vi "resultsColumnsSamplingInfo.vi"(10 "chValuesIn":string[](array[string]), 11 "chNamesIn":string[](array[string])) -> (2 "chValuesOut":string[](array[string]), 3 "chNamesOut":string[](array[string]))   [LabVIEW 2021]
uses:
  Globals/Meas_global.vi
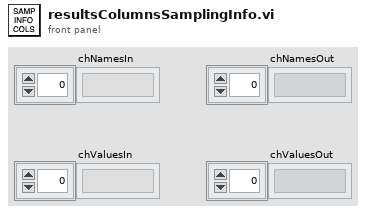
[diagram p1: front panel]
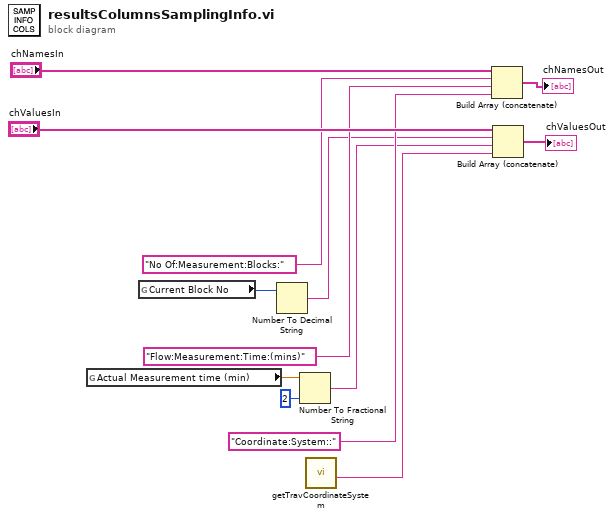
[diagram p0: block diagram]
diagram:
  n1 = global read "Meas_global.vi" "Actual Measurement time (min)"() -> (w3:dbl)
  n2 = global read "Meas_global.vi" "Current Block No"() -> (w9:i32)
  n3 = Number To Decimal String(number=w9) -> (decimal integer string=w4:string)  [unwired: 1 out]
  n4 = Number To Fractional String(number=w3, precision (6)=i16 2) -> (F-format string=w1:string)  [unwired: 2 out]
  n5 = call "getTravCoordinateSystem.vi"() -> ("coordName"=w8:string)  [unwired: 10 in, 1 out]
  n6 = Build Array (concatenate)("chNamesIn", "No Of:Measurement:Blocks:", "Flow:Measurement:Time:(mins)", "Coordinate:System::") -> (→"chNamesOut":string[])
  n7 = Build Array (concatenate)("chValuesIn", w4, w1, w8) -> (→"chValuesOut":string[])
